vi "Subtractive Colour Mixer.vi"(8 "error in (no error)":errorcluster, 11 "Colours":u32[](array[colorbox])) -> (0 "error out":errorcluster, 3 "Mixed colour":u32(colorbox)=16777216)   [LabVIEW 2018, in "Colour Lab.lvlib"]
uses:
  Colour Lab.lvlib
  Colour to RGB.vi
  RGB to CMYK.vi
  RGB to Colour.vi
  CMYK to RGB.vi
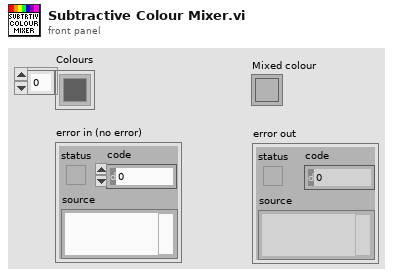
[diagram p1: front panel]
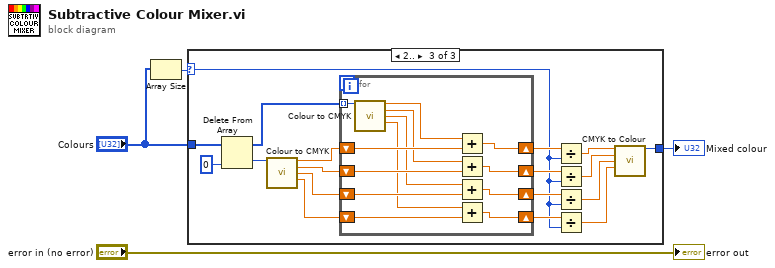
[diagram p0: block diagram]
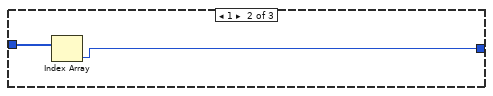
[diagram p3: hidden frame]
diagram:
  n1 = Array Size(array="Colours") -> (size(s)=w2:i32)
  n2 = case shown="2.." w2 {
    selector: w2 -> [_ _ w7]
    tunnel: "Colours" -> [_ w6 w22]
    tunnel: [_ w5 w16] -> w1
    frame ..0 {
    }
    frame 1 {
      n3 = Index Array(array=w6) -> (element=w5:u32)  [unwired: 1 in]
    }
    frame 2.. {
      n4 = Delete From Array(array=w22, index=0) -> (deleted portion=w21:u32, array with subset deleted=w23:u32[])  [unwired: 1 in]
      n5 = call "Colour to CMYK.vi"("Colour"=w21) -> ("Cyan(%)"=w20:dbl, "Magenta(%)"=w19:dbl, "Yellow(%)"=w18:dbl, "Key/Black(%)"=w17:dbl)  [unwired: 9 in, 2 out]
      n6 = for {
        shift-right: [w32] -> w15
        shift-left: w20 -> [w34]
        tunnel: w23 -> [w37] mode=indexing
        shift-right: [w33] -> w14
        shift-left: w19 -> [w35]
        shift-right: [w28] -> w13
        shift-left: w18 -> [w36]
        shift-right: [w25] -> w12
        shift-left: w17 -> [w27]
        n7 = call "Colour to CMYK.vi"("Colour"=w37) -> ("Cyan(%)"=w29:dbl, "Magenta(%)"=w30:dbl, "Yellow(%)"=w31:dbl, "Key/Black(%)"=w26:dbl)  [unwired: 9 in, 2 out]
        n8 = Add(x=w29, y=w34) -> (x+y=w32:dbl)
        n9 = Add(x=w30, y=w35) -> (x+y=w33:dbl)
        n10 = Add(x=w31, y=w36) -> (x+y=w28:dbl)
        n11 = Add(x=w26, y=w27) -> (x+y=w25:dbl)
      }
      n12 = Divide(x=w15, y=w7) -> (x/y=w11:dbl)
      n13 = Divide(x=w14, y=w7) -> (x/y=w10:dbl)
      n14 = Divide(x=w13, y=w7) -> (x/y=w9:dbl)
      n15 = Divide(x=w12, y=w7) -> (x/y=w8:dbl)
      n16 = call "CMYK to Colour.vi"("Cyan(%)"=w11, "Magenta(%)"=w10, "Yellow(%)"=w9, "Key/Black(%)"=w8) -> ("Colour"=w16:u32)  [unwired: 10 in, 1 out]
    }
  }
  "Mixed colour" <- w1
  "error out" <- "error in (no error)"
